vi "ClsLoadConfig.vi"(8 "error in (no error)":errorcluster, 11 "XML File Path":path) -> (0 "error out":errorcluster, 2 "ClsCondigureValues (Array)":string[](array[string]), 3 "ClsConfigureValues (Cluster)":T1)   [LabVIEW 2015]
uses:
  TypeDefs/ClsConfigureValues.ctl
  TypeDefs/ClsCommandOrder.ctl
  <vilib>/Utility/xml.llb/Read From XML File(string).vi
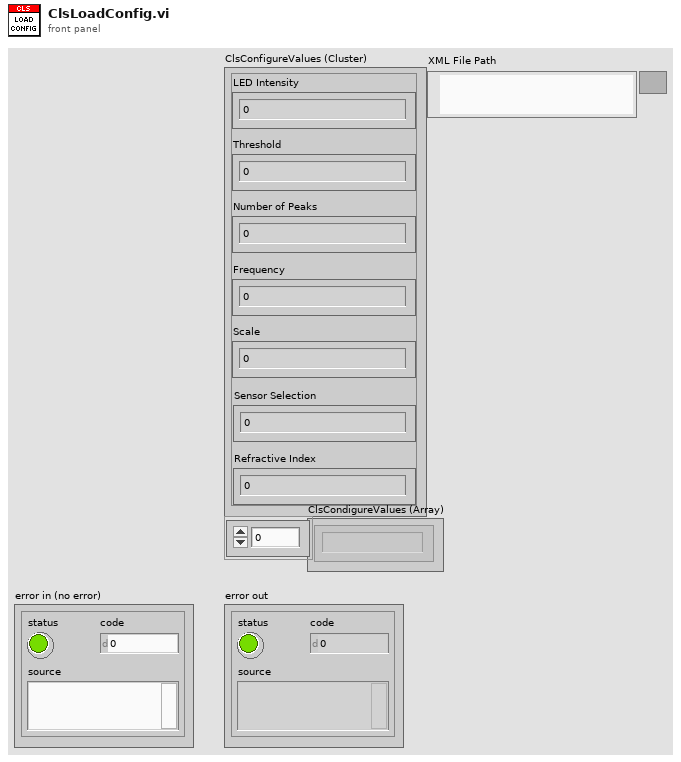
[diagram p1: front panel]
types:
  T1 = typedef "ClsConfigureValues.ctl" = cluster{"LED Intensity":dbl, "Threshold":dbl, "Number of Peaks":dbl, "Frequency":dbl, "Scale":dbl, "Sensor Selection":dbl, "Refractive Index":dbl}
  T2 = typedef "ClsCommandOrder.ctl" = string[]
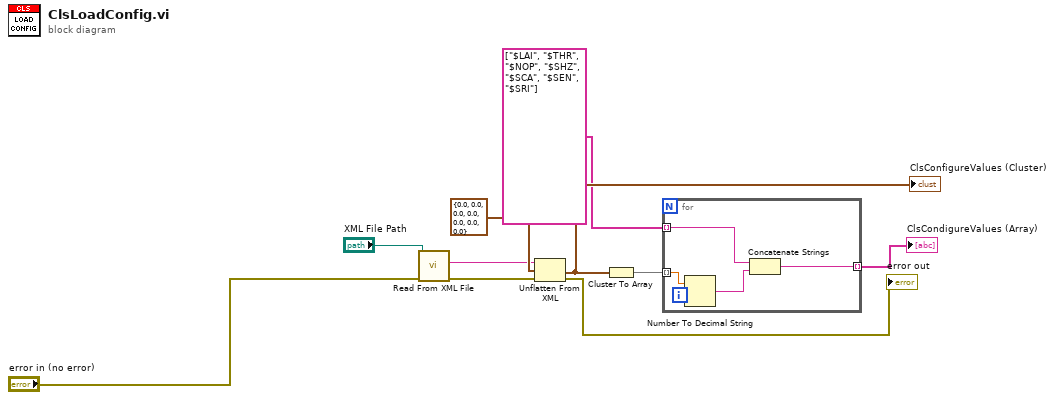
[diagram p0: block diagram]
diagram:
  n1 = call-poly <vilib>:"Read From XML File.vi"("error in (no error)"="error in (no error)", "XML File Path"="XML File Path") -> ("error out"=w5:errorcluster, "XML Elements"=w4:string)  [unwired: 7 in, 1 out]
  n2 = Unflatten From XML(xml string=w4, type=T1 {"LED Intensity"=0.0, "Threshold"=0.0, "Number of Peaks"=0.0, "Frequency"=0.0, "Scale"=0.0, "Sensor Selection"=0.0, "Refractive Index"=0.0} ("ClsConfigureValues"), error in (no error)=w5) -> (value=w10:T1, error out=→"error out":errorcluster)
  "ClsConfigureValues (Cluster)" <- w10
  n3 = Cluster To Array(cluster=w10) -> (array=w7:dbl[])
  n4 = for {
    tunnel: T2 ["$LAI", "$THR", "$NOP", "$SHZ", "$SCA", "$SEN", "$SRI"] ("InitCommandArray") -> [w14] mode=indexing
    tunnel: w7 -> [w13] mode=indexing
    tunnel: [w11] -> w8 mode=indexing
    n5 = Number To Decimal String(number=w13) -> (decimal integer string=w12:string)  [unwired: 1 in]
    n6 = Concatenate Strings(w14, w12) -> (w11:string)
  }
  "ClsCondigureValues (Array)" <- w8
